vi "9.GyropMove.vi"() -> ()   [LabVIEW 2017]
uses:
  <vilib>/Platform/TimedLoop/XDataNode/timing_clust.ctl
  <vilib>/Platform/TimedLoop/XDataNode/nitl_modes.ctl
  <vilib>/Platform/TimedLoop/XDataNode/wakeup.ctl
  <vilib>/Platform/TimedLoop/XDataNode/XDataNode.xnode
  <vilib>/addons/control/pid/pid.llb/PID (DBL).vi
  <vilib>/Platform/TimedLoop/XDataNode/XDNodeRunTimeDep.lvlib
  <vilib>/addons/control/pid/NI_PID_pid.lvlib
panel:
  out "角度比较":cluster{"期望旋转角度":dbl, "转动的角度":dbl}(graph)
  in  "期望旋转角度":dbl format="%.2f"
  in  "PID参数":T1={"proportional gain (Kc)"=1.0, "integral time (Ti, min)"=0.01, "derivative time (Td, min)"=0.0} caption="PID增益" {"derivative time (Td, min)" format="%.3f"; "integral time (Ti, min)" format="%.3f"; "proportional gain (Kc)" format="%.3f"}
  out "实际转动的角度":dbl caption="转动的角度" format="%0.2f"
  in  "error in (no error)":errorcluster
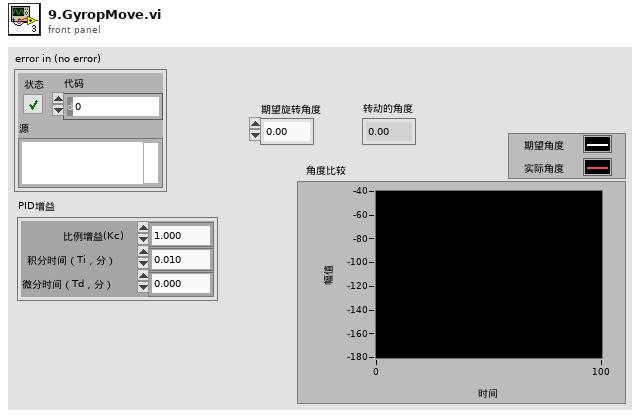
[diagram p1: front panel]
types:
  T1 = cluster{"proportional gain (Kc)":dbl, "integral time (Ti, min)":dbl, "derivative time (Td, min)":dbl}
  T2 = typedef "XDNodeRunTimeDep.lvlib/timing_clust.ctl" = cluster{"Expected End [f-1]":u64, "Actual End [f-1]":u64, "Finished Late? [f-1]":bool, "Expected End [i-1]":u64, "Actual End [i-1]":u64, "Finished Late? [i-1]":bool, "Expected Start [i]":u64, "Actual Start [i]":u64, "Expected Start [f]":u64, "Actual Start [f]":u64, "Source Name":string, "Structure Name":string, "Period":i64, "Deadline":i64, "Offset":i64, "Start":i64, "Priority":i32, "Timeout":i32, "Mode":T3, "Wakeup Reason":T4, "Error":errorcluster, "Source Type":string, "Secondary Source Type":string, "Global End Time":u64, "Global Start Time":u64, "Frame Duration":u64, "Iteration Duration":u64, "Assigned CPU":i32, "I/O Scan Engine Mode":u32}
  T3 = typedef "XDNodeRunTimeDep.lvlib/nitl_modes.ctl" = enum32{"No Change", "Process missed periods, maintain original phase", "Discard missed periods, maintain original phase", "Process missed periods, ignore original phase", "Discard missed periods, ignore original phase"}
  T4 = typedef "XDNodeRunTimeDep.lvlib/wakeup.ctl" = enum32{"Normal", "Aborted", "Asynchronous wakeup", "Timing source error", "Timed loop error", "Timeout"}
  T5 = typedef "I2C.lvlib/I2C Reference.ctl" = cluster{"myRIO Reference":T6, "I2C Channels Enum":T10, "I2C Configuration":T11}
  T6 = typedef "myRIO Generic Hardware Reference.ctl" = cluster{"myRIO Model":T7, "myRIO Hardware Reference":T8}
  T7 = typedef "Hardware Version Enum.ctl" = enum16{"Unknown", "myRIO-1900", "myRIO-1950", "roboRIO", "NI ELVIS RIO CM"}
  T8 = typedef "myRIO v1.0 Reference.ctl" = cluster{"Generic FPGA Reference":T9, "Allow multiple opens":bool}
  T9 = typedef "Generic FPGA Reference.ctl" = refnum<k20>
  T10 = typedef "I2C Channels Enum.ctl" = enum16{"Not Connected", "A/I2C", "B/I2C", "I2C/I2C"}
  T11 = typedef "I2C.lvlib/I2C Configuration.ctl" = cluster{"I2C Transfer Rate":T12}
  T12 = typedef "I2C.lvlib/I2C Transfer Rate.ctl" = enum16{"Standard mode (100 kbps)", "Fast mode (400 kbps)"}
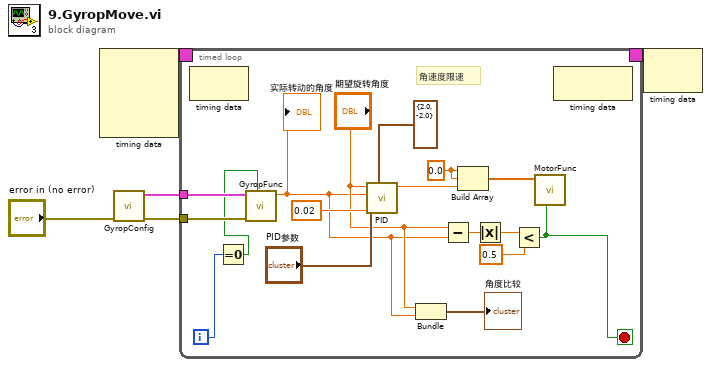
[diagram p0: block diagram]
diagram:
  n1 = node-c288() -> (w5:T2)  [unwired: 4 in]
  n2 = call "GyropConfig.vi"("error in (no error)"="error in (no error)") -> ("error out"=w2:errorcluster, "I2C对象的引用"=w1:T5)  [unwired: 9 in]
  n3 = timed-loop {
    timing: w5 -> [_]
    timing-out: [_] -> w4
    tunnel: w2 -> [w21]
    tunnel: w1 -> [w22]
    i -> [w20]
    stop <- w9 stop-if-true
    w14 = 0.0 ("元素")
    # "角速度限速"
    n4 = node-c288() -> ()  [unwired: 1 in, 1 out]
    n5 = Equal To 0?(x=w20) -> (x = 0?=w19:bool)
    n6 = call "GyropFunc.vi"("重置积分器"=w19, "error in (no error)"=w21, "I2C Ref In"=w22) -> ("转动的角度"=w7:dbl)  [unwired: 6 in, 1 out]
    "实际转动的角度" <- w7
    n7 = call-poly <vilib>:"PID.vi"("output range"=cluster{"output high":dbl, "output low":dbl} {"output high"=2.0, "output low"=-2.0}, "dt (s)"=0.02, "PID gains"="PID参数", "process variable"=w7, "setpoint"="期望旋转角度") -> ("output"=w15:dbl)  [unwired: 5 in, 1 out]
    n8 = Bundle("期望旋转角度"="期望旋转角度", "转动的角度"=w7) -> (→"角度比较":cluster{"期望旋转角度":dbl, "转动的角度":dbl})  [unwired: 1 in]
    n9 = Subtract(x="期望旋转角度", y=w7) -> (x-y=w12:dbl)
    n10 = Build Array(w14, w14, w15) -> (w13:dbl[])
    n11 = Absolute Value(x=w12) -> (abs(x)=w11:dbl)
    n12 = Less?(x=w11, y=0.5) -> (x < y?=w9:bool)
    n13 = call "MotorFunc.vi"("停止"=w9, "把当前坐标系下期望小\n车在X、Y、θ的速度作\n为逆运算的输入"=w13) -> ()  [unwired: 8 in, 2 out]
    n14 = node-c288() -> ()  [unwired: 1 in, 1 out]
  }
  n15 = node-c288(w4) -> ()  [unwired: 1 out]
